vi "initialize.vi"(0 "HGF_SVVarManVisitor_delete":refnum<class "HGF_SVVarManVisitor_delete.lvclass">, 3 "initializationData":variant, 5 "error in (no error)":errorcluster, 7 "binaryString":string, 8 "I8 Array":i8[](array[numeric]), 9 "prependSize? (T)":bool, 11 "byteOrder (0:big-endian, network order)":T1(ring)) -> (14 "dup HGF_SVVarManVisitor_delete":refnum<class "HGF_SVVarManVisitor_delete.lvclass">, 17 "found?":bool, 19 "error out":errorcluster)   [LabVIEW 2012, in "HGF_SV.lvlib" / "HGF_SVVarManVisitor_delete.lvclass"]
doc: "This is a dynamic dispatch VI to be implemented by child classes to initialize their attributes.\n\n<B>Recommendation:</B> Use Variant for initialization data."
uses:
  HGF_SVVarManVisitor_delete.lvclass
  HGF_BaseClasses/HGF_Visitor/HGF_Visitor.lvclass
  HGF_SVVarManVisitor_delete.lvclass/HGF_SVVarManVisitor_delete.ctl
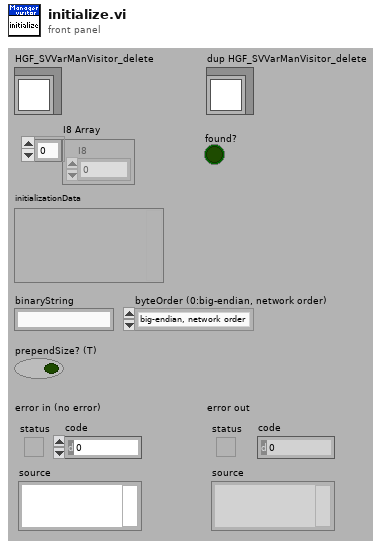
[diagram p1: front panel]
types:
  T1 = enum16{"big-endian, network order", "native, host order", "little-endian"}
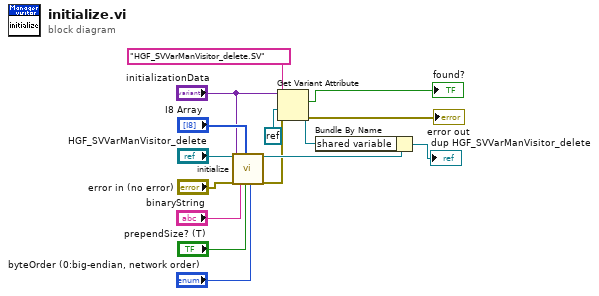
[diagram p0: block diagram]
diagram:
  n1 = call-parent "initialize.vi"("HGF_Visitor"="HGF_SVVarManVisitor_delete", "initializationData"="initializationData", "error in (no error)"="error in (no error)", "binaryString"="binaryString", "I8 Array"="I8 Array", "prependSize? (T)"="prependSize? (T)", "byteOrder (0:big-endian, network order)"="byteOrder (0:big-endian, network order)") -> ("dup HGF_Visitor"=w9:refnum<class "HGF_SVVarManVisitor_delete.lvclass">, "error out"=w4:errorcluster)  [unwired: 10 in, 1 out]
  n2 = Get Variant Attribute(Variant="initializationData", name="HGF_SVVarManVisitor_delete.SV", default value (empty Variant)=refnum<k21> refnum, error in=w4) -> (found=→"found?":bool, value=w1:refnum<k21>, error out=→"error out":errorcluster)  [unwired: 1 out]
  n3 = Bundle By Name(cluster=w9, "shared variable"=w1) -> (→"dup HGF_SVVarManVisitor_delete":refnum<class "HGF_SVVarManVisitor_delete.lvclass">)
